vi "11b-async.vi"() -> ()   [LabVIEW 2018, in "LV2Julia_examples.lvlib"]
uses:
  LV2Julia_examples.lvlib
  LV2Julia_core/VIs/Server or client state.ctl
  LV2Julia_core/VIs/detailed error info.ctl
  LV2Julia_core/VIs/StackFrame.ctl
  LV2Julia_core/VIs/Commands.ctl
  be4745b6-8471-45fc-b8a0-8968ce92ea4b.vi
  877f6708-f4bd-42a3-8abe-32eb8c2c970e.vi
  be4745b6-8471-45fc-b8a0-8968ce92ea4b.vi/01ce1741-ea78-47f8-98ed-e79163fb1a9b.vi
  877f6708-f4bd-42a3-8abe-32eb8c2c970e.vi/896d20f1-cb1d-4420-8f1f-f93355f5adea.vi
  be4745b6-8471-45fc-b8a0-8968ce92ea4b.vi/01ce1741-ea78-47f8-98ed-e79163fb1a9b.vi/cc3cf2af-bc3b-4fb6-855b-7562c4d0bfeb.vi
  be4745b6-8471-45fc-b8a0-8968ce92ea4b.vi/01ce1741-ea78-47f8-98ed-e79163fb1a9b.vi/c77cecd8-10de-4d46-bc1c-57302a887fda.vi
  be4745b6-8471-45fc-b8a0-8968ce92ea4b.vi/01ce1741-ea78-47f8-98ed-e79163fb1a9b.vi/2cafb1dd-d397-4b79-911a-06d102936120.vi
  877f6708-f4bd-42a3-8abe-32eb8c2c970e.vi/896d20f1-cb1d-4420-8f1f-f93355f5adea.vi/9892c125-836d-426b-b144-8af50d50507b.vi
  877f6708-f4bd-42a3-8abe-32eb8c2c970e.vi/896d20f1-cb1d-4420-8f1f-f93355f5adea.vi/80aac079-9052-42cf-b2c3-c29da6bba58d.vi
  877f6708-f4bd-42a3-8abe-32eb8c2c970e.vi/896d20f1-cb1d-4420-8f1f-f93355f5adea.vi/6d5e1d21-cb4d-4981-8d16-85d9352ac501.vi
  LV2Julia_core/VIs/jl-scripts path.vi
  LV2Julia_core/VIs/check ID validity.vi
  LV2Julia_core/VIs/bindata_descr to JSON.vi
  LV2Julia_core/VIs/check cluster field names.vi
  LV2Julia_core/VIs/concat JSON.vi
  LV2Julia_core/VIs/build request.vi
  LV2Julia_core/VIs/Parse server response.vi
  LV2Julia_core/VIs/log jl exceptions.vi
  LV2Julia_core/LV2Julia_core.lvlib
panel:
  out "notif 2":bool
  out "Boolean":bool
  out "notification":bool
  in  "stop polling":bool
  out "stopping":bool
  out "done":bool
  out "ticket":i32
  in  "summands":cluster{"x":dbl, "y":dbl}={"x"=2.0, "y"=2.0}
  in  "next":bool
  out "x+y":dbl=nan
  out "detailed error info":T1
  out "current error":errorcluster
  out "final error":errorcluster
  out "short err code":u8
  in  "stop":bool
  out "ZMQ timeout":bool
  out "Julia script file path":path
  out "temporary script path":path
  out "Jl Server state":T3
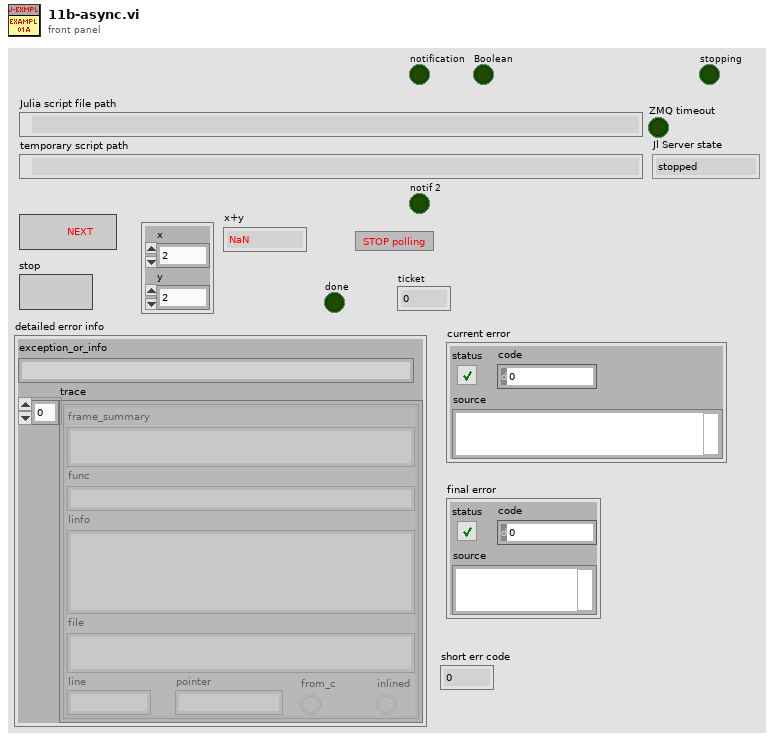
[diagram p1: front panel]
types:
  T1 = typedef "LV2Julia_core.lvlib/detailed error info.ctl" = cluster{"exception_or_info":string, "trace":T2[]}
  T2 = typedef "LV2Julia_core.lvlib/StackFrame.ctl" = cluster{"frame_summary":string, "func":string, "linfo":string, "file":string, "line":i32, "pointer":u64, "from_c":bool, "inlined":bool}
  T3 = typedef "LV2Julia_core.lvlib/Server or client state.ctl" = enum16{"stopped", "running", "unknown"}
  T4 = typedef "LV2Julia_core.lvlib/Commands.ctl" = enum16{"Start Jl-server & Init LV-client", "Send request & Get response ", "Stop Jl-server & Cleanup LV-client", "Cleanup LV-client", "Start Jl-server", "Stop Jl-server", "Init LV-Client", "Cleanup LV-Client", "(not allowed)", "Set LV Client state", "Set Jl Server state", "set ZMQ timeout", "read ZMQ timeout", "read-out state"}
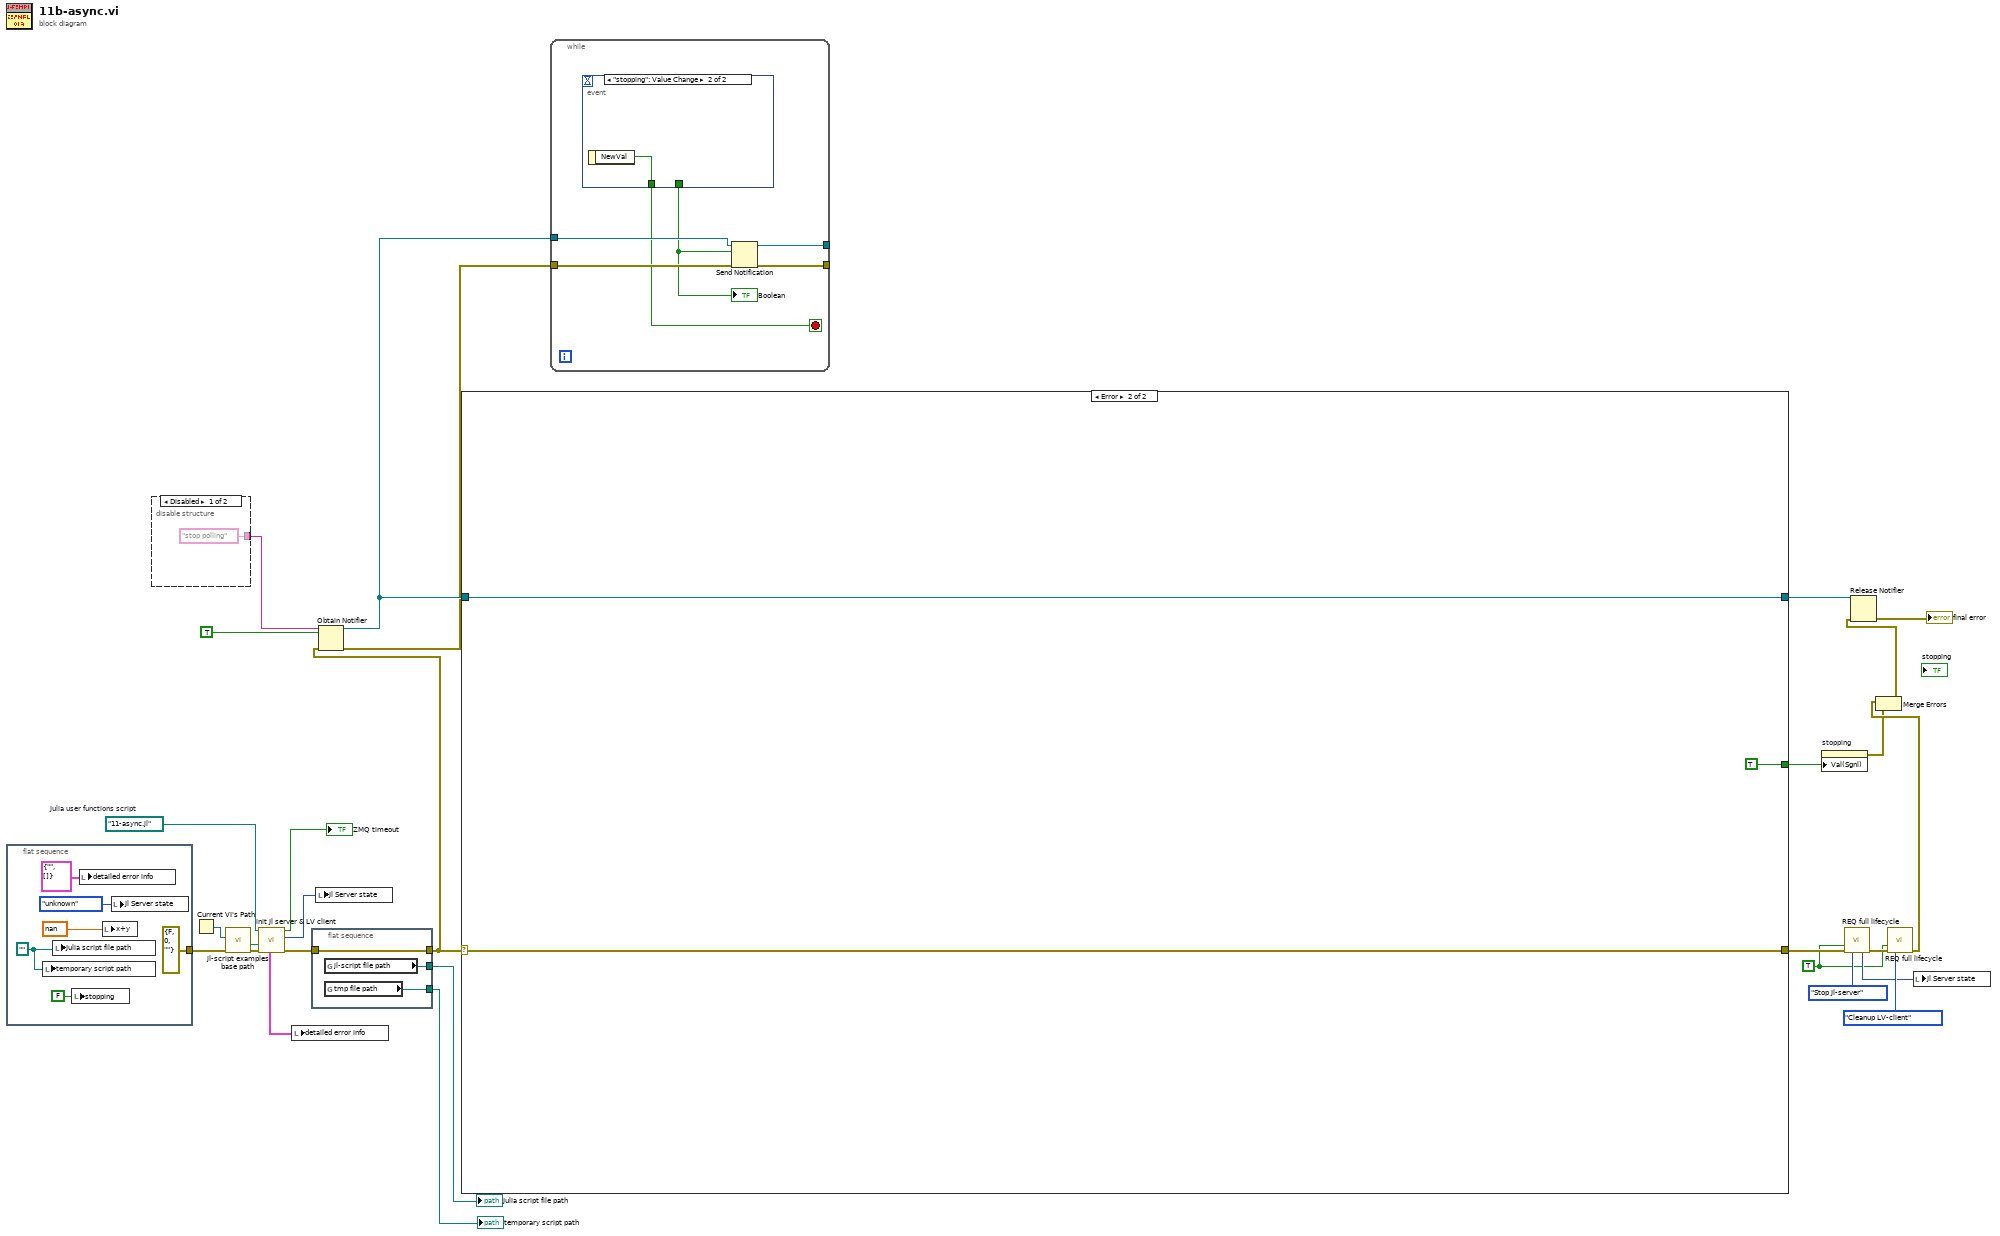
[diagram p0: block diagram]
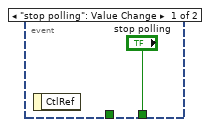
[diagram p3: hidden frame]
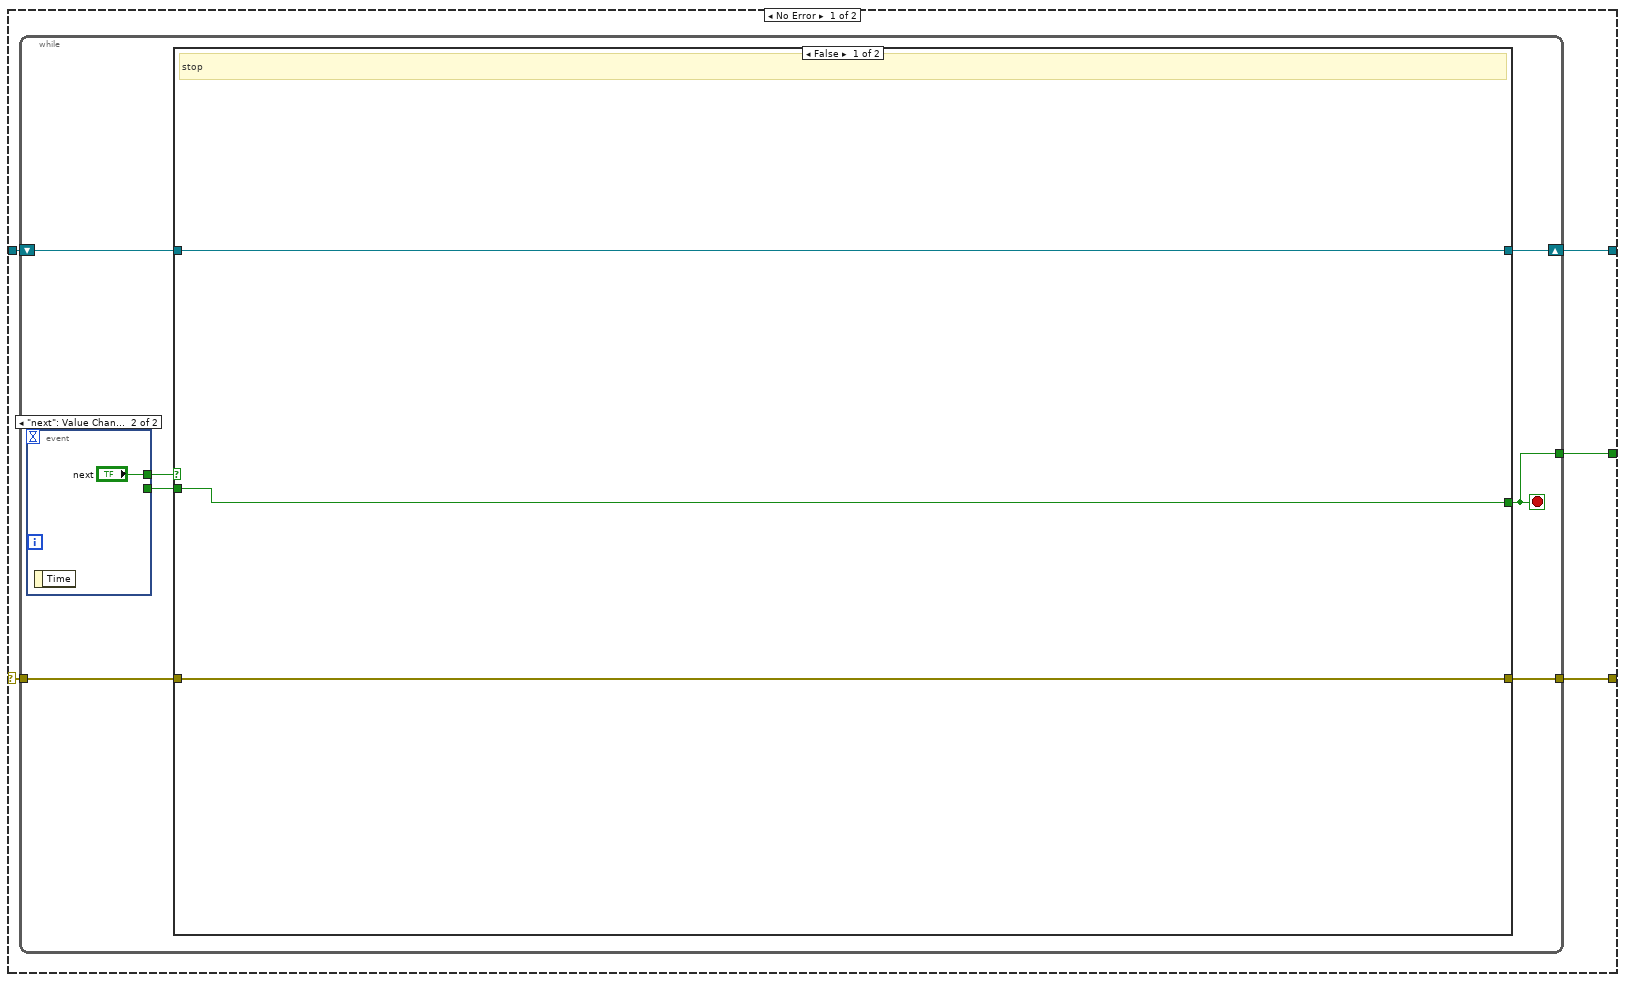
[diagram p4: hidden frame]
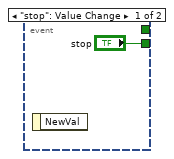
[diagram p5: hidden frame]
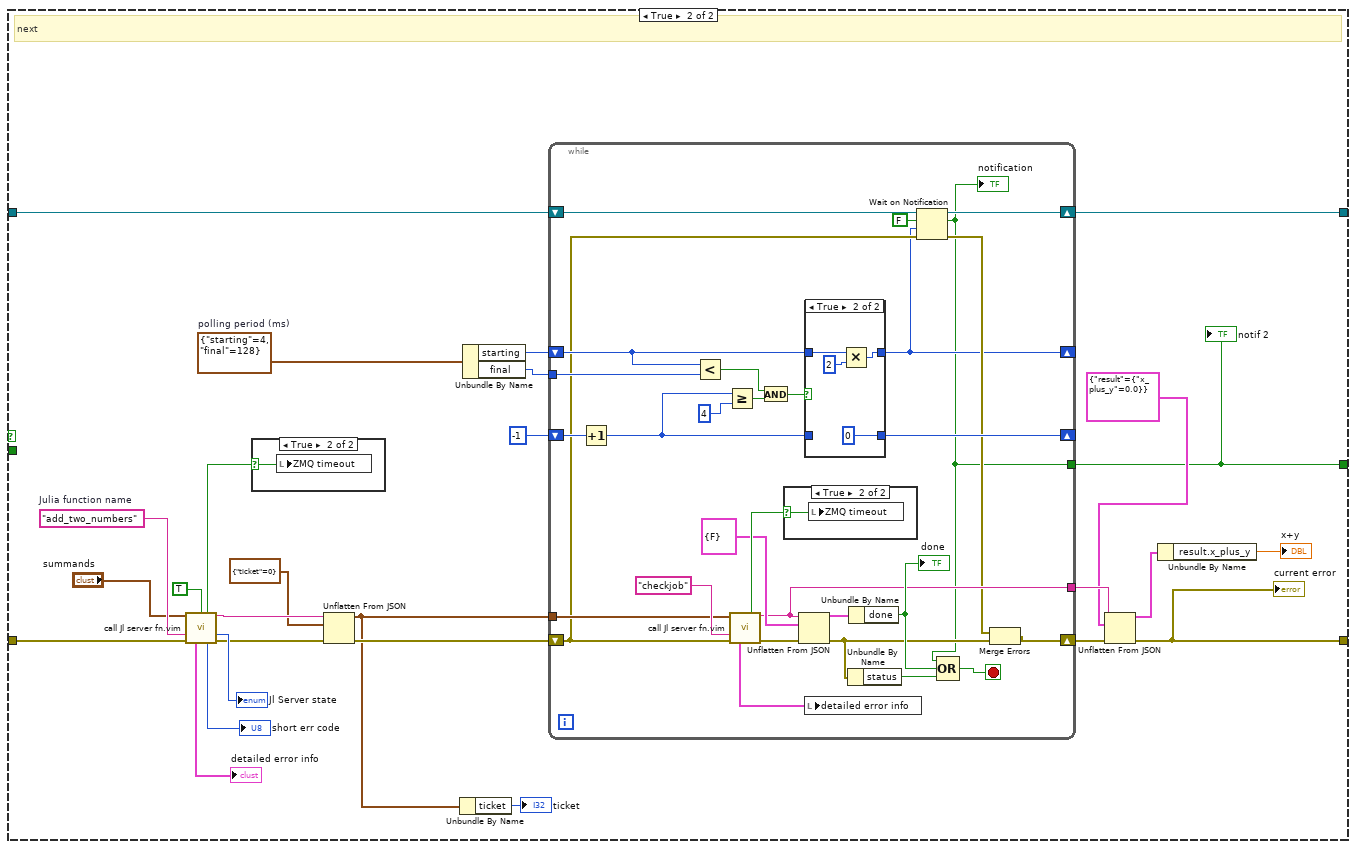
[diagram p6: hidden frame]
diagram:
  w21 = path "11-async.jl"  # Julia user functions script
  w5 = TRUE ("Force command")
  n1 = flat-sequence {
    tunnel: [errorcluster {"status"=FALSE, "code"=0, "source"=""} ("error in (no error)")] -> w17
    frame #0 {
      w30 = path ""
      n2 = local write "temporary script path"(w30) -> ()
      n3 = local write "Julia script file path"(w30) -> ()
      n4 = local write "stopping"(FALSE ("stopping")) -> ()
      n5 = local write "detailed error info"(T1 {"exception_or_info"="", "trace"=[]} ("detailed error info")) -> ()
      n6 = local write "x+y"(nan ("Server response")) -> ()
      n7 = local write "Jl Server state"(Server_or_client_state."unknown" ("Jl Server state out")) -> ()
    }
  }
  n8 = disable-structure shown="Disabled" {
    disable-tunnel: ["stop polling" ("name (unnamed)") _] -> w11
    frame Disabled {
    }
    frame Enabled {
    }
  }
  n9 = Current VI's Path() -> (path=w14:path)
  n10 = call "jl-script examples base path.vi"("error in (no error)"=w17, "calling example VI path"=w14) -> ("error out"=w16:errorcluster, "jl-script-examples base path"=w15:path)  [unwired: 8 in]
  n11 = call "init Jl server & LV client.vi"("error in (no error)"=w16, "Base path (not a path)"=w15, "Julia user functions script"=w21) -> ("error out"=w19:errorcluster, "Jl Server state out"=w18:T3, "timeout?"=→"ZMQ timeout":bool, "detailed error info"=w13:T1)  [unwired: 3 in, 2 out]
  n12 = local write "detailed error info"(w13) -> ()
  n13 = flat-sequence {
    tunnel: [w38] -> w9
    tunnel: w19 -> [w38]
    tunnel: [w37] -> w23
    tunnel: [w36] -> w24
    frame #0 {
      n14 = global read "jl-scripts path.vi" "jl-script file path"() -> (w37:path)
      n15 = global read "jl-scripts path.vi" "tmp file path"() -> (w36:path)
    }
  }
  n16 = local write "Jl Server state"(w18) -> ()
  n17 = Obtain Notifier(name (unnamed)=w11, notification data type=TRUE, error in (no error)=w9) -> (notifier out=w10:refnum<notifier>, error out=w8:errorcluster)  [unwired: 1 in, 1 out]
  n18 = case shown="Error" w9 {
    selector: w9 -> [w42 w122]
    tunnel: [w43 w122] -> w28
    tunnel: w10 -> [w41 w121]
    tunnel: [w40 w121] -> w7
    tunnel: [w39 TRUE ("stop")] -> w1
    frame No Error {
      n19 = while {
        tunnel: w42 -> [w49]
        tunnel: [w50] -> w43
        shift-right: [w45] -> w40
        shift-left: w41 -> [w46]
        tunnel: [w44] -> w39
        stop <- w44 stop-if-true
        n20 = event shown="[1] \"next\": Value Change" {
          selector: _ -> [_ _]
          dyn-events: _ -> [_ _]
          timeout: _ -> [_ _]
          tunnel: [_ "next"] -> w48
          tunnel: ["stop" _] -> w47
          event "stop": Value Change {
            n21 = event-data() -> ()  [unwired: 1 in, 1 out]
          }
          event "next": Value Change {
            n22 = event-data() -> ()  [unwired: 1 in, 1 out]
          }
        }
        n23 = case shown="False" w48 {
          tunnel: [w53 w73] -> w50
          tunnel: w49 -> [w53 w75]
          tunnel: [w54 w56] -> w44
          tunnel: w47 -> [w54 _]
          tunnel: w46 -> [w55 w58]
          tunnel: [w55 w57] -> w45
          frame False {
            # "stop"
          }
          frame True {
            w62 = cluster{"starting":i32, "final":i32} {"starting"=4, "final"=128}  # polling period (ms)
            w81 = "add_two_numbers"  # Julia function name
            # "next"
            n24 = call "call Jl server fn.vim"("Arguments 1"="summands", "async call (false)"=TRUE ("timeout?"), "fun2call"=w81, "error in (no error)"=w75) -> ("timeout?"=w78:bool, "JSON received"=w71:string, "Jl Server state out"=→"Jl Server state":T3, "detailed error info"=→"detailed error info":T1, "return code"=→"short err code":u8, "error out"=w70:errorcluster)  [unwired: 5 in, 1 out]
            n25 = case shown="True" w78 {
              selector: w78 -> [_ w119]
              frame False {
              }
              frame True {
                n26 = local write "ZMQ timeout"(w119) -> ()
              }
            }
            n27 = Unflatten From JSON(JSON string=w71, type and defaults=cluster{"ticket":i32} {"ticket"=0} ("parsed response"), error in (no error)=w70) -> (value=w67:cluster{"ticket":i32}, error out=w68:errorcluster)  [unwired: 4 in]
            n28 = Unbundle By Name(w67) -> ("ticket"=→"ticket":i32)
            n29 = Unbundle By Name(w62) -> ("starting"=w61:i32, "final"=w59:i32)
            n30 = while {
              tunnel: w67 -> [w110]
              tunnel: [w104] -> w65
              shift-right: [w88] -> w64
              shift-left: w68 -> [w89]
              shift-right: [w85] -> _
              shift-left: w61 -> [w93]
              shift-right: [w98] -> _
              shift-left: -1 ("counter") -> [w99]
              tunnel: w59 -> [w95]
              shift-right: [w86] -> w57
              shift-left: w58 -> [w90]
              tunnel: [w84] -> w56
              stop <- w102 stop-if-true
              n31 = Increment(x=w99) -> (x+1=w92:i32)
              n32 = Less?(x=w93, y=w95) -> (x < y?=w94:bool)
              n33 = Greater Or Equal?(x=w92, y=4) -> (x >= y?=w96:bool)
              n34 = call "call Jl server fn.vim"("Arguments 1"=w110, "fun2call"="checkjob" ("Julia function name"), "error in (no error)"=w89) -> ("timeout?"=w109:bool, "JSON received"=w104:string, "detailed error info"=w100:T1, "error out"=w108:errorcluster)  [unwired: 6 in, 3 out]
              n35 = And(x=w94, y=w96) -> (x .and. y?=w91:bool)
              n36 = case shown="True" w109 {
                selector: w109 -> [_ w118]
                frame False {
                }
                frame True {
                  n37 = local write "ZMQ timeout"(w118) -> ()
                }
              }
              n38 = Unflatten From JSON(JSON string=w104, type and defaults=cluster{"done":bool} {"done"=FALSE}, error in (no error)=w108) -> (value=w106:cluster{"done":bool}, error out=w103:errorcluster)  [unwired: 4 in]
              n39 = case shown="True" w91 {
                tunnel: w92 -> [w113 _]
                tunnel: [w113 0] -> w98
                tunnel: w93 -> [w112 w116]
                tunnel: [w112 w115] -> w85
                frame False {
                }
                frame True {
                  n40 = Multiply(x=w116, y=2) -> (x*y=w115:i32)
                }
              }
              n41 = local write "detailed error info"(w100) -> ()
              n42 = Unbundle By Name(w103) -> ("status"=w101:bool)
              n43 = Unbundle By Name(w106) -> ("done"=w105:bool)
              "done" <- w105
              n44 = Wait on Notification(notifier=w90, ignore previous (F)=FALSE, timeout in ms (-1)=w85, error in (no error)=w89) -> (notifier out=w86:refnum<notifier>, notification=w84:bool, error out=w87:errorcluster)  [unwired: 1 out]
              "notification" <- w84
              n45 = Compound Arithmetic op=OR(w84, w105, w101) -> (w102:bool)
              n46 = Merge Errors(w87, w103) -> (w88:errorcluster)
            }
            "notif 2" <- w56
            n47 = Unflatten From JSON(JSON string=w65, type and defaults=cluster{"result":cluster{"x_plus_y":dbl}} {"result"={"x_plus_y"=0.0}}, error in (no error)=w64) -> (value=w74:cluster{"result":cluster{"x_plus_y":dbl}}, error out=w73:errorcluster)  [unwired: 4 in]
            "current error" <- w73
            n48 = Unbundle By Name(w74) -> ("result.x_plus_y"=→"x+y":dbl)
          }
        }
      }
    }
    frame Error {
    }
  }
  n49 = while {
    tunnel: w10 -> [w128]
    tunnel: [w127] -> _
    tunnel: w8 -> [w126]
    tunnel: [w125] -> _
    stop <- w123 stop-if-true
    n50 = event shown="[1] \"stopping\": Value Change" {
      selector: _ -> [_ _]
      dyn-events: _ -> [_ _]
      timeout: _ -> [_ _]
      tunnel: ["stop polling" _] -> w124
      tunnel: [_ w130] -> w123
      event "stop polling": Value Change {
        n51 = event-data() -> ()  [unwired: 1 in, 1 out]
      }
      event "stopping": Value Change {
        n52 = event-data() -> ("NewVal"=w130:bool)  [unwired: 1 in]
      }
    }
    "Boolean" <- w124
    n53 = Send Notification(notification=w124, notifier=w128, error in (no error)=w126) -> (notifier out=w127:refnum<notifier>, error out=w125:errorcluster)
  }
  n54 = property on="stopping" class="Bool (strict)"("Val(Sgnl)"=w1) -> (error out=w2:errorcluster)  [unwired: 2 in, 1 out]
  n55 = call "REQ full lifecycle.vi"("Force command"=w5, "error in"=w28, "command"=Commands."Stop Jl-server") -> ("Jl Server state out"=w22:T3, "error out"=w26:errorcluster)  [unwired: 6 in, 5 out]
  n56 = call "REQ full lifecycle.vi"("Force command"=w5, "error in"=w26, "command"=Commands."Cleanup LV-client") -> ("error out"=w4:errorcluster)  [unwired: 6 in, 6 out]
  n57 = Merge Errors(w4, w2) -> (w3:errorcluster)
  n58 = Release Notifier(notifier=w7, error in (no error)=w3) -> (error out=→"final error":errorcluster)  [unwired: 1 in, 2 out]
  n59 = local write "Jl Server state"(w22) -> ()
  "temporary script path" <- w24
  "Julia script file path" <- w23
